vi "Get Report Type.vi"(0 "report in":refnum<class "NI_report.lvclass">, 11 "error in (no error)":errorcluster) -> (4 "report out":refnum<class "NI_report.lvclass">, 8 "report type":T1(ring)=enum."HTML", 15 "error out":errorcluster)   [LabVIEW 2020, in "NI_report.lvclass"]
doc: "This VI is deprecated. Use the following VI instead:\n\nvi.lib\\Utility\\NIReport.llb\\Report Type.vi\n\nReturns the report type, such as standard on Windows, or HTML on all platforms, of a specified report.\n\nThis VI also returns Microsoft Word or Excel report types."
uses:
  NI_report.lvclass
panel:
  # "This VI is deprecated. Use the following VI instead:\n\nvi.lib\\Utility\\NIReport.llb\\Report Type.vi"
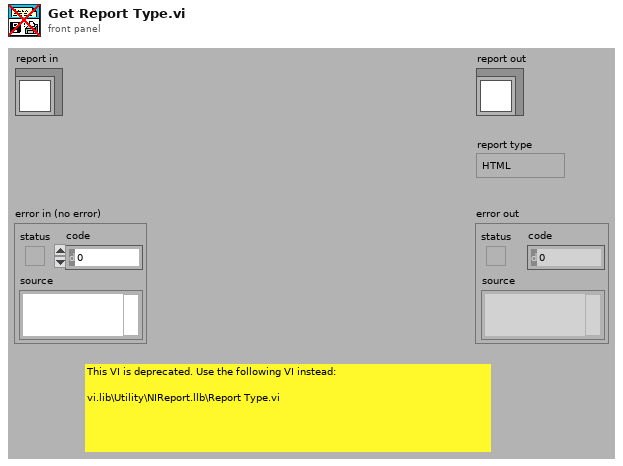
[diagram p1: front panel]
types:
  T1 = enum16{"Standard Report", "HTML", "Word", "Excel"}
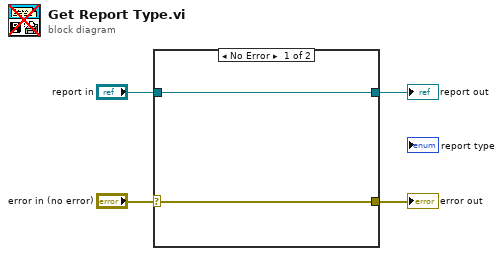
[diagram p0: block diagram]
diagram:
  n1 = case shown="No Error" "error in (no error)" {
    selector: "error in (no error)" -> [w6 w8]
    tunnel: [w6 w8] -> w3
    tunnel: [w5 w7] -> w1
    tunnel: "report in" -> [w5 w7]
    frame No Error {
    }
    frame Error {
    }
  }
  "error out" <- w3
  "report out" <- w1
